vi "Quick release working.vi"() -> ()   [LabVIEW 2018]
doc: "The myRIO Project template acquires acceleration data from the onboard accelerometer and displays the changes of acceleration values in a waveform chart."
uses:
  <vilib>/myRIO/Common/Instrument Driver Framework/myRIO v1.0/UART/vis/myRIO v1.0 Close UART.vi
  <vilib>/myRIO/Common/Instrument Driver Framework/Utilities/vis/FPGA Ref Manager.vi
  <vilib>/myRIO/Common/Instrument Driver Framework/myRIO v1.0/myRIO v1.0 Reset FPGA.vi
  <vilib>/myRIO/Common/Instrument Driver Framework/myRIO v1.0/IRQ/vis/myRIO v1.0 IRQ Info FGV.vi
  <vilib>/myRIO/Common/Instrument Driver Framework/myRIO v1.0/IRQ/vis/myRIO v1.0 Timer IRQ Info FGV.vi
  <vilib>/myRIO/Common/Instrument Driver Framework/myRIO v1.0/IRQ/vis/myRIO v1.0 ISR Agent.vi
  <vilib>/myRIO/Instrument Drivers/Utilities/Utilities.lvlib
panel:
  in  "Channel Names":tag[](array[tag])=["A/DIO0", "A/DIO1"]
  in  "Stop":bool
  in  "Deploy / Retract [T/F]":bool
  out "error out 2":errorcluster
  in  "Stop 2":bool
  # "DIO3\nDIO4"
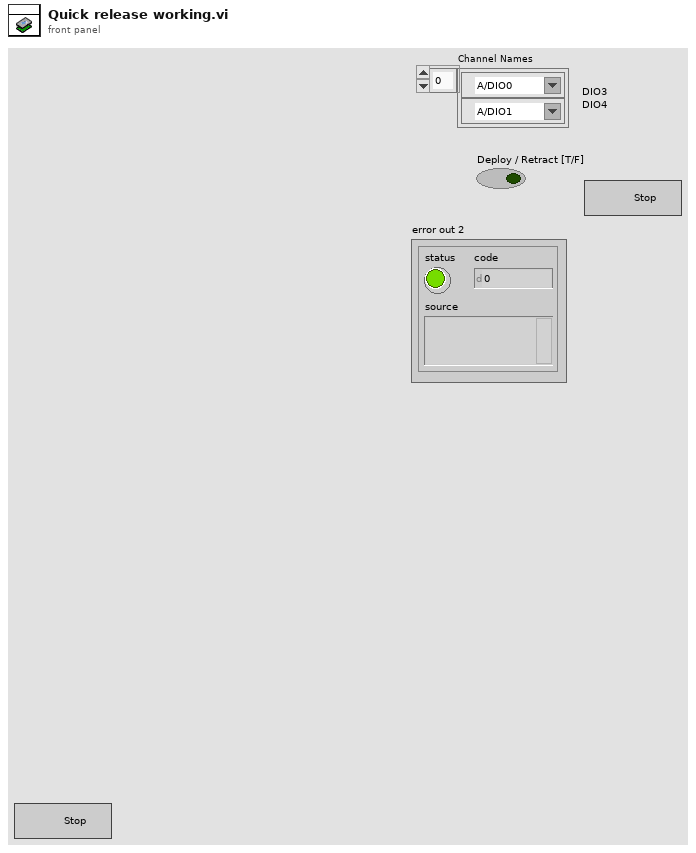
[diagram p1: front panel]
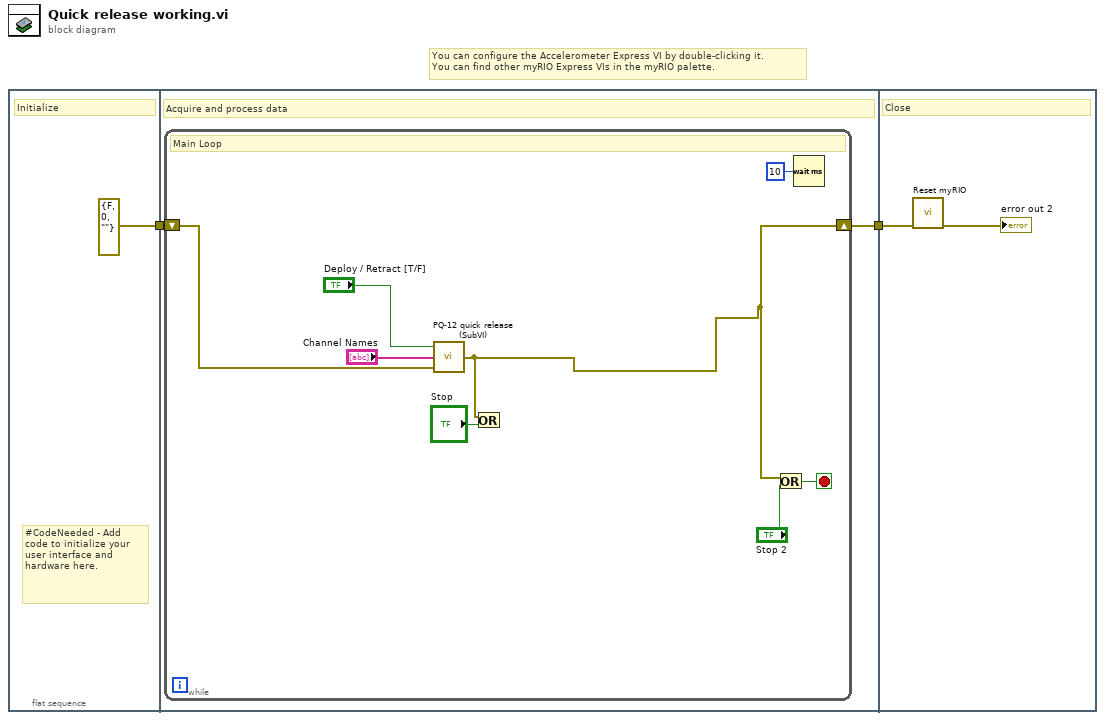
[diagram p0: block diagram]
diagram:
  # "You can configure the Accelerometer Express VI by double-clicking it.\nYou can find other myRIO Express VIs in the myRIO palette."
  n1 = flat-sequence {
    tunnel: [errorcluster {"status"=FALSE, "code"=0, "source"=""} ("error in (no error)")] -> w2
    tunnel: w2 -> [w5]
    tunnel: [w4] -> w1
    tunnel: w1 -> [w15]
    frame #0 {
      # "#CodeNeeded - Add code to initialize your user interface and hardware here."
      # "Initialize"
    }
    frame #1 {
      # "Acquire and process data"
      n2 = while {
        shift-right: [w7] -> w4
        shift-left: w5 -> [w8]
        stop <- w12 stop-if-true
        # "Main Loop"
        n3 = call "PQ-12 quick release (SubVI).vi"("error in (no error)"=w8, "Channel Names"="Channel Names", "Deploy / Retract [T/F]"="Deploy / Retract [T/F]") -> ("error out"=w7:errorcluster)
        n4 = Or(x=w7, y="Stop") -> ()  [unwired: 1 out]
        n5 = Or(x=w7, y="Stop 2") -> (x .or. y?=w12:bool)
        n6 = Wait (ms)(milliseconds to wait=u32 10) -> ()  [unwired: 1 out]
      }
    }
    frame #2 {
      # "Close"
      n7 = call <vilib>:"Reset myRIO.vi"("error in (no error)"=w15) -> ("error out"=→"error out 2":errorcluster)  [unwired: 10 in]
    }
  }
